vi "Quad Ctr, Index Save.vi"() -> ()   [LabVIEW 2015]
doc: "This VI interprets a quadrature encoder signal and asynchronously saves the current position value on every valid index state. A valid index state is defined when Line A, Line B and Input Z are all low.\n\nThe 16 bit Position uses hardware lines A and B of the quadrature encoder. Input Z is linked to SWITCH1 on the sbRIO evaluation board."
uses:
  <vilib>/Platform/TimedLoop/XDataNode/timing_clust.ctl
  <vilib>/Platform/TimedLoop/XDataNode/nitl_modes.ctl
  <vilib>/Platform/TimedLoop/XDataNode/wakeup.ctl
  <vilib>/rvi/Emulation/niFpgaSctlEmulationGetInTimedLoop.vi
  <vilib>/rvi/Emulation/niFpgaEmulationReportErrorSimple.vi
  <vilib>/rvi/Emulation/niFpgaGetClockAttributes.vi
  <vilib>/rvi/Emulation/niFpgaCriticalErrorInLSC.vi
  <vilib>/rvi/eio/common/nirviEmuTemplateMethod_errors.vi
  <vilib>/Platform/TimedLoop/XDataNode/XDataNode.xnode
  <vilib>/eio/EIONode/EIONode.xnode
  <vilib>/Platform/TimedLoop/XDataNode/XDNodeRunTimeDep.lvlib
panel:
  in  "stop":bool
  out "16 bit Position":i16
  out "Index Save":i16
  # "This VI interprets a quadrature encoder signal and asynchronously\nsaves the current position value on every valid index state.  A valid \nindex state is defined when Line A, Line B and Input Z are all low.\n\nThe 16 bit Position uses hardware lines A and B of the quadrature \nencoder. Input Z is linked to PB1 on the LabVIEW RIO evaluation board."
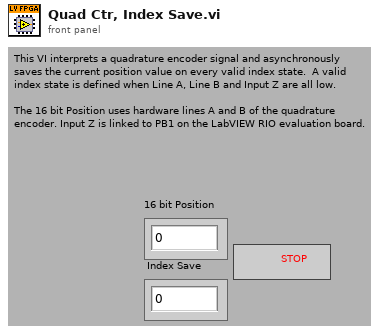
[diagram p1: front panel]
types:
  T1 = typedef "XDNodeRunTimeDep.lvlib/timing_clust.ctl" = cluster{"Expected End [f-1]":u64, "Actual End [f-1]":u64, "Finished Late? [f-1]":bool, "Expected End [i-1]":u64, "Actual End [i-1]":u64, "Finished Late? [i-1]":bool, "Expected Start [i]":u64, "Actual Start [i]":u64, "Expected Start [f]":u64, "Actual Start [f]":u64, "Source Name":string, "Structure Name":string, "Period":i64, "Deadline":i64, "Offset":i64, "Start":i64, "Priority":i32, "Timeout":i32, "Mode":T2, "Wakeup Reason":T3, "Error":errorcluster, "Source Type":string, "Secondary Source Type":string, "Global End Time":u64, "Global Start Time":u64, "Frame Duration":u64, "Iteration Duration":u64, "Assigned CPU":i32, "I/O Scan Engine Mode":u32}
  T2 = typedef "XDNodeRunTimeDep.lvlib/nitl_modes.ctl" = enum32{"No Change", "Process missed periods, maintain original phase", "Discard missed periods, maintain original phase", "Process missed periods, ignore original phase", "Discard missed periods, ignore original phase"}
  T3 = typedef "XDNodeRunTimeDep.lvlib/wakeup.ctl" = enum32{"Normal", "Aborted", "Asynchronous wakeup", "Timing source error", "Timed loop error", "Timeout"}
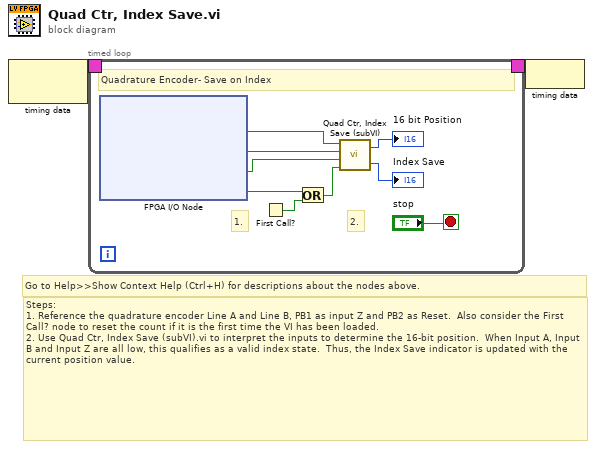
[diagram p0: block diagram]
diagram:
  # "Go to Help>>Show Context Help (Ctrl+H) for descriptions about the nodes above."
  # "Steps:\n1. Reference the quadrature encoder Line A and Line B, PB1 as input Z and PB2 as Reset.  Also consider the First Call? node to reset the count if it is the first time the VI has been loaded.\n2. Use Quad Ctr, Index Save (subVI).vi to interpret the inputs to determine the 16-bit position.  When Input A, Input B and Input Z are all low, this qualifies as a valid index state.  Thus, the Index Save indicator is updated with the current position value."
  n1 = node-c288() -> (w2:T1)  [unwired: 1 out]
  n2 = timed-loop {
    timing: w2 -> [_]
    timing-out: [_] -> w1
    stop <- "stop" stop-if-true
    # "2."
    # "1."
    # "Quadrature Encoder- Save on Index"
    n3 = xnode "FPGA I/O Node"() -> ("ENCODER CH.A"=w10:bool, "ENCODER CH.B"=w9:bool, "PB1"=w8:bool, "PB2"=w4:bool)  [unwired: 4 in, 4 out]
    n4 = First Call?() -> (First Call?: T/F=w3:bool)
    n5 = Or(x=w4, y=w3) -> (x .or. y?=w5:bool)
    n6 = call "Quad Ctr, Index Save (subVI).vi"("Reset"=w5, "Input Z"=w8, "Input B"=w9, "Input A"=w10) -> ("Index Save"=→"Index Save":i16, "16 bit Position"=→"16 bit Position":i16)
  }
  n7 = node-c288(w1) -> ()
